vi "NotificationBar.vi"(9 "NotificationBarString":string) -> ()   [LabVIEW 2014]
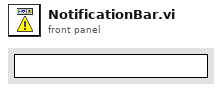
[diagram p1: front panel]
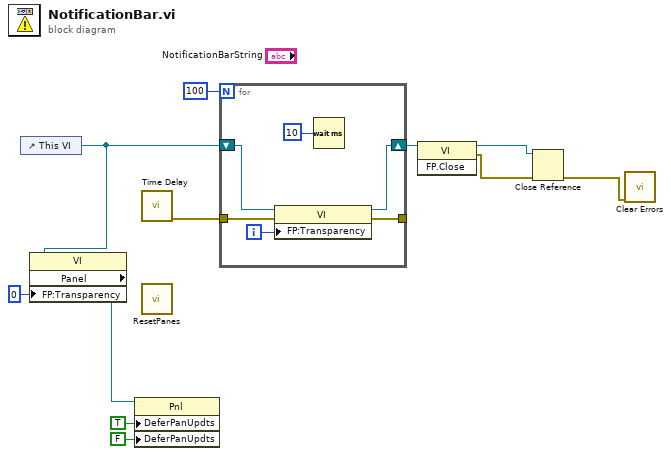
[diagram p0: block diagram]
diagram:
  n1 = control-ref of="This VI"() -> (w5:refnum<vi>)
  n2 = property class="VI"(reference=w5, "FP:Transparency"=u8 0 ("Front Panel Window:Transparency")) -> ("Panel"=w4:refnum<vi>)  [unwired: 1 in, 2 out]
  n3 = property class="Pnl"(reference=w4, "DeferPanUpdts"=TRUE ("Defer Panel Updates"), "DeferPanUpdts"=FALSE ("Defer Panel Updates")) -> ()  [unwired: 1 in, 2 out]
  n4 = call "Time Delay"() -> ("error out"=w9:errorcluster)  [unwired: 11 in]
  n5 = call "ResetPanes.vi"() -> ()  [unwired: 12 in]
  n6 = for {
    N: 100 -> [_]
    tunnel: w9 -> [w14]
    shift-right: [w13] -> w10
    shift-left: w5 -> [w17]
    tunnel: [w12] -> _
    i -> [w16]
    n7 = property class="VI"(reference=w17, error in=w14, "FP:Transparency"=w16) -> (reference out=w13:refnum<vi>, error out=w12:errorcluster)
    n8 = Wait (ms)(milliseconds to wait=u32 10) -> ()  [unwired: 1 out]
  }
  n9 = invoke class="VI" method="FP.Close"(reference=w10) -> (reference out=w8:refnum<vi>, error out=w7:errorcluster)  [unwired: 2 in, 1 out]
  n10 = Close Reference(reference=w8, error in (no error)=w7) -> (error out=w6:errorcluster)
  n11 = call <vilib>:"Clear Errors.vi"("error in (no error)"=w6) -> ()  [unwired: 5 in, 2 out]
